vi "hardware_initialize_hardware.vi"(8 "error in (no error)":errorcluster, 11 "galvo in":refnum<class "galvo.lvclass">) -> (0 "error out":errorcluster, 3 "galvo out":refnum<class "galvo.lvclass">)   [LabVIEW 2015, in "galvo.lvclass"]
uses:
  galvo.lvclass
  galvo.lvclass/galvo.ctl
  <vilib>/DAQmx/create/channels.llb/DAQmx Create Channel (AO-Voltage-Basic).vi
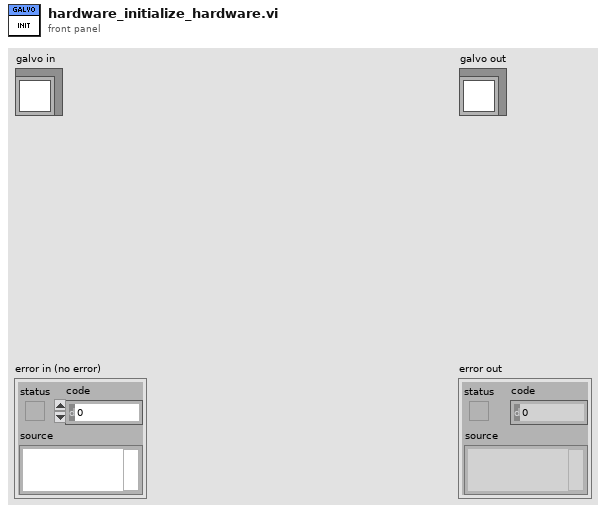
[diagram p1: front panel]
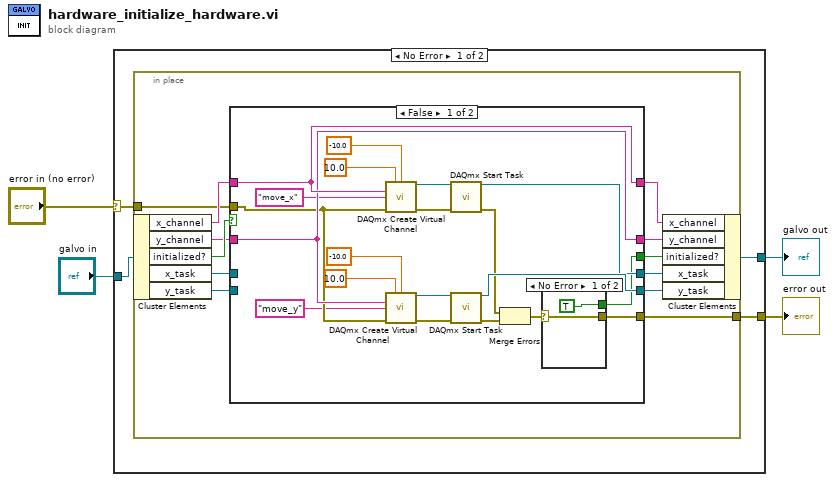
[diagram p0: block diagram]
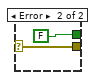
[diagram p2: hidden frame]
diagram:
  n1 = case shown="No Error" "error in (no error)" {
    selector: "error in (no error)" -> [w5 w51]
    tunnel: "galvo in" -> [w8 w52]
    tunnel: [w7 w52] -> w2
    tunnel: [w6 w51] -> w1
    frame No Error {
      n2 = in-place {
        in-place-border: [w10] -> w6
        in-place-border: w5 -> [w9]
        n3 = in-place-cluster #1(w8) -> ("x_channel"=w18:tag, "y_channel"=w17:tag, "initialized?"=w20:bool, "x_task"=w12:refnum<k21>, "y_task"=w11:refnum<k21>)
        n4 = case shown="False" w20 {
          selector: w20 -> [_ w50]
          tunnel: [w22 w50] -> w19
          tunnel: w18 -> [w32 w49]
          tunnel: w17 -> [w31 w48]
          tunnel: [w32 w49] -> w16
          tunnel: [w31 w48] -> w15
          tunnel: [w30 w46] -> w14
          tunnel: [w29 w47] -> w13
          tunnel: w12 -> [_ w47]
          tunnel: w11 -> [_ w46]
          tunnel: [w21 w45] -> w10
          tunnel: w9 -> [w26 w45]
          frame False {
            n5 = call-poly <vilib>:"DAQmx Create Virtual Channel.vi"("maximum value"=10.0, "minimum value"=-10.0, "physical channels"=w32, "name to assign"="move_x", "error in"=w26) -> ("task out"=w38:refnum<k21>, "error out"=w37:errorcluster)  [unwired: 9 in]
            n6 = call-poly <vilib>:"DAQmx Create Virtual Channel.vi"("maximum value"=10.0, "minimum value"=-10.0, "physical channels"=w31, "name to assign"="move_y", "error in"=w26) -> ("task out"=w34:refnum<k21>, "error out"=w33:errorcluster)  [unwired: 9 in]
            n7 = call <vilib>:"DAQmx Start Task.vi"("task/channels in"=w38, "error in"=w37) -> ("task out"=w29:refnum<k21>, "error out"=w28:errorcluster)  [unwired: 12 in]
            n8 = call <vilib>:"DAQmx Start Task.vi"("task/channels in"=w34, "error in"=w33) -> ("task out"=w30:refnum<k21>, "error out"=w27:errorcluster)  [unwired: 12 in]
            n9 = Merge Errors(w28, w27) -> (w23:errorcluster)
            n10 = case shown="No Error" w23 {
              selector: w23 -> [w41 w43]
              tunnel: [TRUE FALSE] -> w22
              tunnel: [w41 w43] -> w21
              frame No Error {
              }
              frame Error {
              }
            }
          }
          frame True {
          }
        }
        n11 = in-place-cluster #1("x_channel"=w16, "y_channel"=w15, "initialized?"=w19, "x_task"=w13, "y_task"=w14) -> (w7:refnum<class "galvo.lvclass">)
      }
    }
    frame Error {
    }
  }
  "error out" <- w1
  "galvo out" <- w2
